vi "Launch.vi"(8 "error in (no error)":errorcluster, 10 "Show Front Panel? (F)":bool, 11 "API-Reference in":refnum<k1>) -> (0 "error out":errorcluster, 1 "Already Launched":bool, 3 "API-Reference out":refnum<k1>)   [LabVIEW 2018, in "Copy of Actor.lvclass"]
uses:
  Copy of Actor.lvclass
  API-Data.ctl
  Stopped.ctl
  Event-References.ctl
  Stop.ctl
  Launched.ctl
  Some Request.ctl
  Some Response.ctl
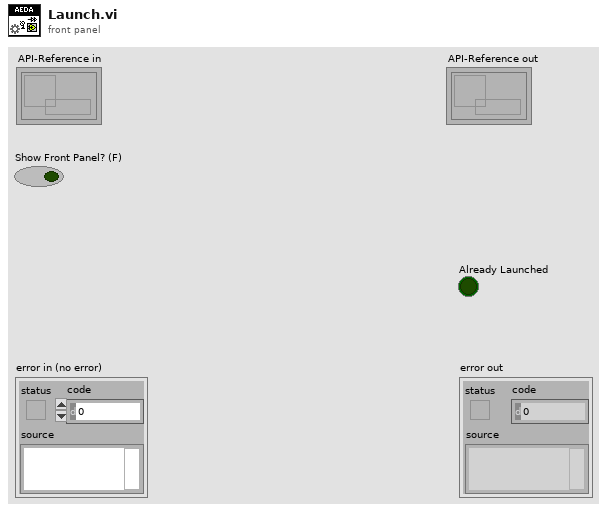
[diagram p1: front panel]
types:
  T1 = typedef "Copy of Actor.lvclass/API-Data.ctl" = cluster{"Launch":refnum<notifier>, "Stopped":refnum<user-event>, "Actor-Events":T2, "Stopped Registration":refnum<event-registration>}
  T2 = typedef "Copy of Actor.lvclass/Event-References.ctl" = cluster{"Stop":refnum<user-event>, "Launched":refnum<user-event>, "Some Request":refnum<user-event>}
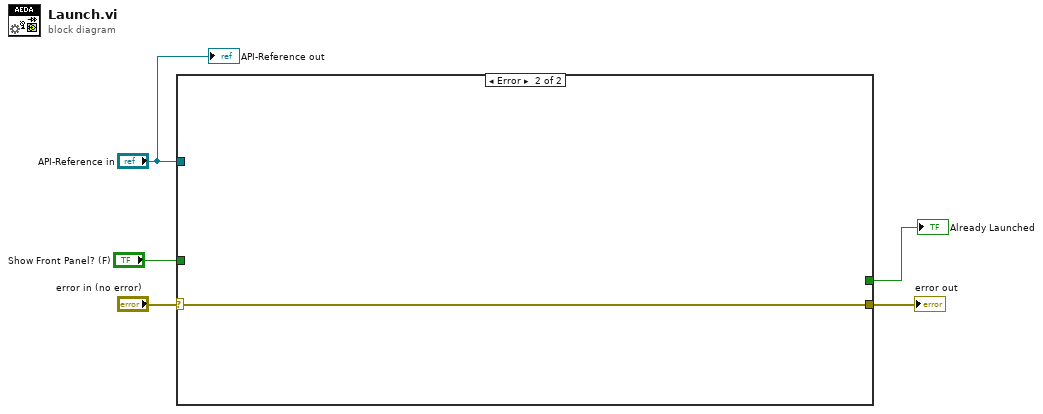
[diagram p0: block diagram]
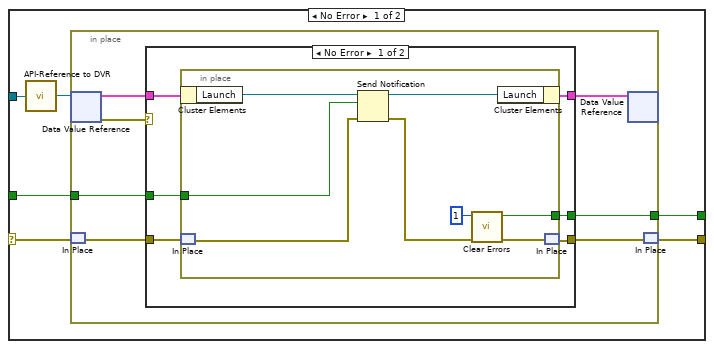
[diagram p2: hidden frame]
diagram:
  n1 = case shown="Error" "error in (no error)" {
    selector: "error in (no error)" -> [w11 w35]
    tunnel: [w10 w35] -> w4
    tunnel: "API-Reference in" -> [w7 _]
    tunnel: [w9 _] -> w3
    tunnel: "Show Front Panel? (F)" -> [w8 _]
    frame No Error {
      n2 = call "API-Reference to DVR.vi"("API-Reference in"=w7) -> ("Data Value Reference out"=w6:refnum<data-value>)
      n3 = in-place {
        in-place-border: [w13] -> w9
        in-place-border: w8 -> [w12]
        n4 = in-place-dvr #1(w6) -> (w17:T1, w18:errorcluster)
        n5 = in-place-match #2(w11) -> (w15:errorcluster)
        n6 = case shown="No Error" w18 {
          selector: w18 -> [_ w34]
          tunnel: w17 -> [w20 w33]
          tunnel: [w19 w33] -> w16
          tunnel: w15 -> [w24 _]
          tunnel: [w23 w34] -> w14
          tunnel: [w22 _] -> w13
          tunnel: w12 -> [w21 _]
          frame No Error {
            n7 = in-place {
              in-place-border: [w27] -> w22
              in-place-border: w21 -> [w26]
              n8 = in-place-cluster #3(w20) -> ("Launch"=w25:refnum<notifier>)
              n9 = in-place-match #4(w24) -> (w32:errorcluster)
              n10 = Send Notification(notification=w26, notifier=w25, error in (no error)=w32) -> (notifier out=w31:refnum<notifier>, error out=w30:errorcluster)
              n11 = call <vilib>:"Clear Errors.vi"("error in (no error)"=w30, "specific error code to clear (0: all)"=1) -> ("error out"=w29:errorcluster, "specific error cleared?"=w27:bool)  [unwired: 4 in]
              n12 = in-place-cluster #3("Launch"=w31) -> (w19:T1)
              n13 = in-place-match #4(w29) -> (w23:errorcluster)
            }
          }
          frame Error {
          }
        }
        n14 = in-place-dvr #1(w16) -> ()  [unwired: 2 out]
        n15 = in-place-match #2(w14) -> (w10:errorcluster)
      }
    }
    frame Error {
    }
  }
  "error out" <- w4
  "Already Launched" <- w3
  "API-Reference out" <- "API-Reference in"
